vi "toml_file_export.vi"(8 "error in (no error)":errorcluster, 10 "remove comments? (F)":bool, 11 "path in":path) -> (0 "error out":errorcluster, 3 "path out":path)   [LabVIEW 2017]
uses:
  toml_fg_action.ctl
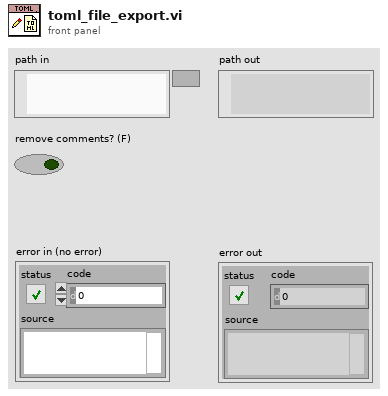
[diagram p1: front panel]
types:
  T1 = typedef "toml_fg_action.ctl" = enum8{"null", "get", "set", "pop", "import", "export", "drop", "sections", "keys", "remove"}
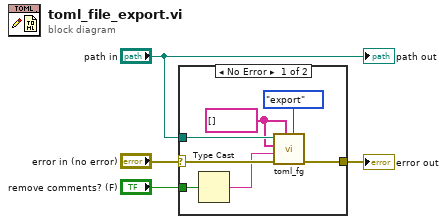
[diagram p0: block diagram]
diagram:
  n1 = case shown="No Error" "error in (no error)" {
    selector: "error in (no error)" -> [w11 w12]
    tunnel: [w10 w12] -> w3
    tunnel: "path in" -> [w9 _]
    tunnel: "remove comments? (F)" -> [w6 _]
    frame No Error {
      w7 = string[] [] ("section")
      n2 = Type Cast(x=w6) -> (*(type *) &x=w5:string)  [unwired: 1 in]
      n3 = call "toml_fg.vi"("action"=toml_fg_action."export", "section"=w7, "error in (no error)"=w11, "value in"=w5, "key"=w7, "path in"=w9) -> ("error out"=w10:errorcluster)  [unwired: 2 in, 3 out]
    }
    frame Error {
    }
  }
  "error out" <- w3
  "path out" <- "path in"
